vi "Read String Camera Status.vi"(8 "error in (no error)":errorcluster, 10 "String Camera Status":string, 11 "Construct String Camera Status in":refnum<class "Construct String Camera Status.lvclass">) -> (0 "error out":errorcluster, 2 "Camera Status":T1, 3 "Construct String Camera Status out":refnum<class "Construct String Camera Status.lvclass">)   [LabVIEW 2018, in "Construct String Camera Status.lvclass"]
doc: "Este VI recebe uma string contendo o status da câmera e retorna um cluster Camera Status."
uses:
  Construct String Camera Status.lvclass
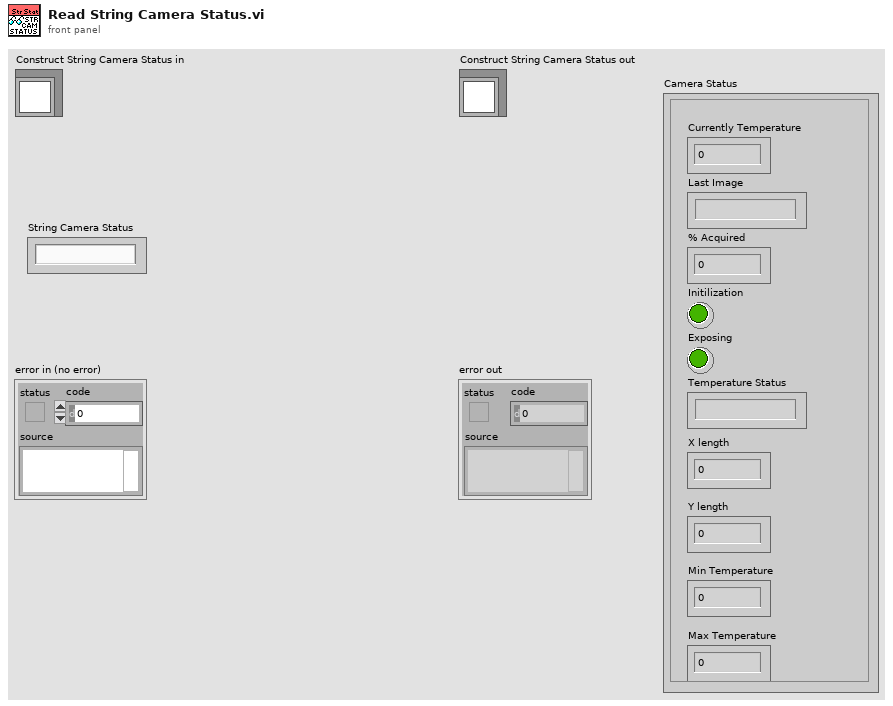
[diagram p1: front panel]
types:
  T1 = cluster{"Currently Temperature":dbl, "Last Image":string, "% Acquired":dbl, "Initilization":bool, "Exposing":bool, "Temperature Status":string, "X length":dbl, "Y length":dbl, "Min Temperature":dbl, "Max Temperature":dbl}
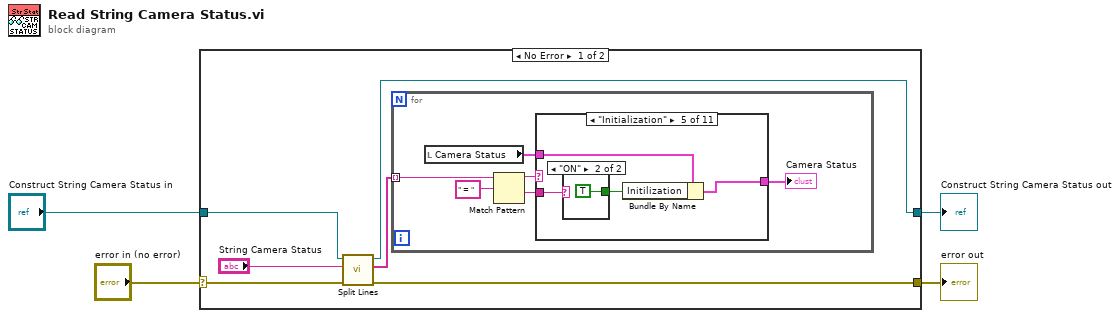
[diagram p0: block diagram]
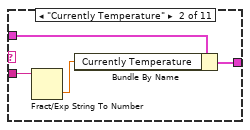
[diagram p3: hidden frame]
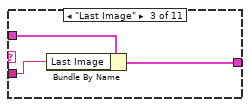
[diagram p4: hidden frame]
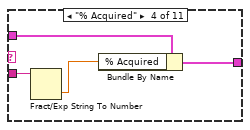
[diagram p5: hidden frame]
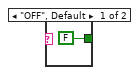
[diagram p6: hidden frame]
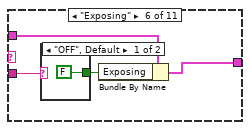
[diagram p7: hidden frame]
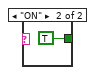
[diagram p8: hidden frame]
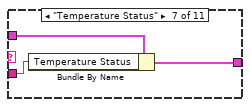
[diagram p9: hidden frame]
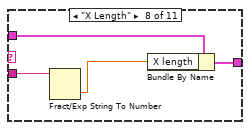
[diagram p10: hidden frame]
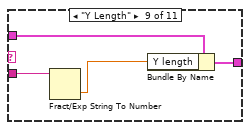
[diagram p11: hidden frame]
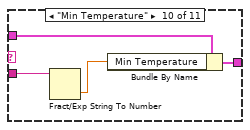
[diagram p12: hidden frame]
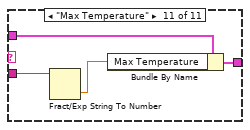
[diagram p13: hidden frame]
diagram:
  n1 = case shown="No Error" "error in (no error)" {
    selector: "error in (no error)" -> [w7 w60]
    tunnel: [w6 w60] -> w4
    tunnel: [w8 w61] -> w2
    tunnel: "Construct String Camera Status in" -> [w9 w61]
    frame No Error {
      n2 = call "Split Lines.vi"("error in"=w7, "String Camera Status"="String Camera Status", "Construct String Camera Status in"=w9) -> ("error out"=w6:errorcluster, "array"=w5:string[], "Construct String Camera Status out"=w8:refnum<class "Construct String Camera Status.lvclass">)  [unwired: 6 in]
      n3 = for {
        tunnel: w5 -> [w16] mode=indexing
        n4 = local read "Camera Status"() -> (w13:T1)
        n5 = Match Pattern(string=w16, regular expression=" = ") -> (before substring=w14:string, after substring=w12:string)  [unwired: 1 in, 2 out]
        n6 = case shown="\"Initialization\"" w14 {
          tunnel: [w17 w21 w24 w28 w32 w38 w43 w47 w51 w55 w59] -> w11
          tunnel: w13 -> [w17 w20 w23 w27 w31 w35 w42 w46 w50 w54 w58]
          tunnel: w12 -> [_ w19 w22 w26 w30 w37 w41 w45 w49 w53 w57]
          frame "False", Default {
          }
          frame "Currently Temperature" {
            n7 = Fract/Exp String To Number(string=w19) -> (number=w18:dbl)  [unwired: 3 in, 1 out]
            n8 = Bundle By Name(cluster=w20, "Currently Temperature"=w18) -> (w21:T1)
          }
          frame "Last Image" {
            n9 = Bundle By Name(cluster=w23, "Last Image"=w22) -> (w24:T1)
          }
          frame "% Acquired" {
            n10 = Fract/Exp String To Number(string=w26) -> (number=w25:dbl)  [unwired: 3 in, 1 out]
            n11 = Bundle By Name(cluster=w27, "% Acquired"=w25) -> (w28:T1)
          }
          frame "Initialization" {
            n12 = case shown="\"ON\"" w30 {
              tunnel: [FALSE TRUE] -> w29
              frame "OFF", Default {
              }
              frame "ON" {
              }
            }
            n13 = Bundle By Name(cluster=w31, "Initilization"=w29) -> (w32:T1)
          }
          frame "Exposing" {
            n14 = case shown="\"OFF\", Default" w37 {
              tunnel: [FALSE TRUE] -> w36
              frame "OFF", Default {
              }
              frame "ON" {
              }
            }
            n15 = Bundle By Name(cluster=w35, "Exposing"=w36) -> (w38:T1)
          }
          frame "Temperature Status" {
            n16 = Bundle By Name(cluster=w42, "Temperature Status"=w41) -> (w43:T1)
          }
          frame "X Length" {
            n17 = Fract/Exp String To Number(string=w45) -> (number=w44:dbl)  [unwired: 3 in, 1 out]
            n18 = Bundle By Name(cluster=w46, "X length"=w44) -> (w47:T1)
          }
          frame "Y Length" {
            n19 = Fract/Exp String To Number(string=w49) -> (number=w48:dbl)  [unwired: 3 in, 1 out]
            n20 = Bundle By Name(cluster=w50, "Y length"=w48) -> (w51:T1)
          }
          frame "Min Temperature" {
            n21 = Fract/Exp String To Number(string=w53) -> (number=w52:dbl)  [unwired: 3 in, 1 out]
            n22 = Bundle By Name(cluster=w54, "Min Temperature"=w52) -> (w55:T1)
          }
          frame "Max Temperature" {
            n23 = Fract/Exp String To Number(string=w57) -> (number=w56:dbl)  [unwired: 3 in, 1 out]
            n24 = Bundle By Name(cluster=w58, "Max Temperature"=w56) -> (w59:T1)
          }
        }
        "Camera Status" <- w11
      }
    }
    frame Error {
    }
  }
  "error out" <- w4
  "Construct String Camera Status out" <- w2
